vi "test Data Width 1 to 64.vi"(8 "error in (no error)":errorcluster, 11 "TestCase in":refnum<class "BCD.lvclass">) -> (0 "error out":errorcluster, 3 "TestCase out":refnum<class "BCD.lvclass">)   [LabVIEW 2027, in "BCD.lvclass"]
uses:
  BCD.lvclass
  080c8e86-f0ef-40bb-bb78-ec3bfa871640.vi
  0459340d-2ef3-43cd-ac4e-b003521538f2.vi
  Source/Get Bits Per Digit from Base.vi
  C:/Program Files/National Instruments/LabVIEW 2027/vi.lib/addons/_JKI Toolkits/VI Tester/TestCase.llb/TestCase.lvclass
  <vilib>/addons/_JKI Toolkits/VI Tester/TestCase.llb/TestCase.lvclass
panel:
  out "BCD encoded value":bool[](array[boolean])
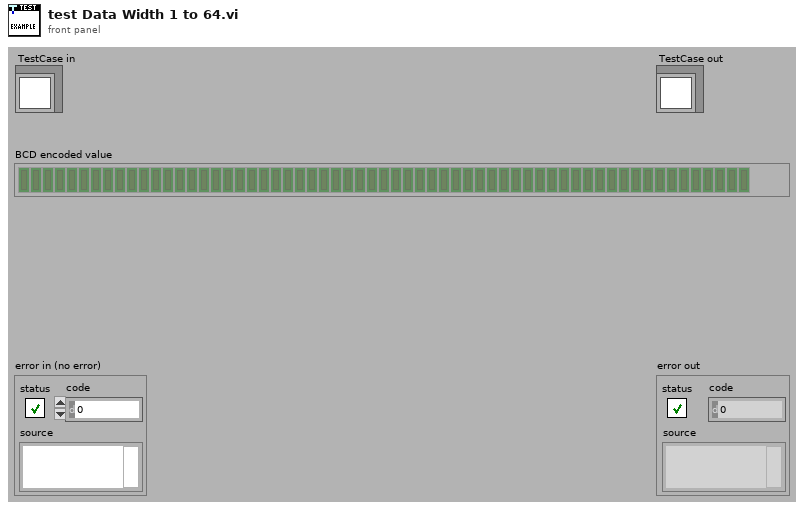
[diagram p1: front panel]
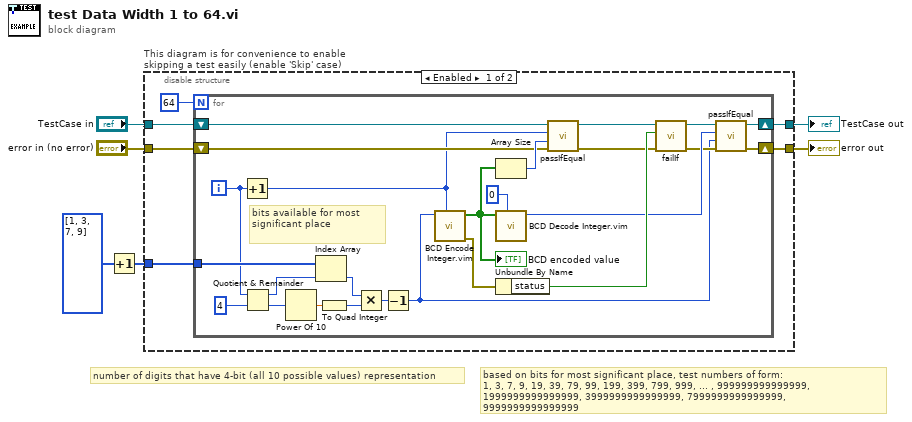
[diagram p0: block diagram]
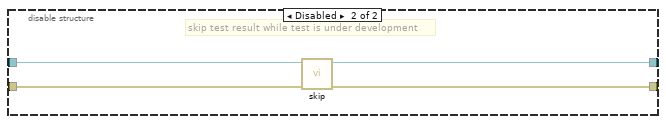
[diagram p2: hidden frame]
diagram:
  # "based on bits for most significant place, test numbers of form:\n1, 3, 7, 9, 19, 39, 79, 99, 199, 399, 799, 999, ... , 999999999999999, \n1999999999999999, 3999999999999999, 7999999999999999, 9999999999999999"
  # "number of digits that have 4-bit (all 10 possible values) representation"
  n1 = Increment(x=i64[] [1, 3, 7, 9]) -> (x+1=w1:i64[])
  n2 = disable-structure "This diagram is for convenience to enable skipping a test easily (enable 'Skip' case)" shown="Enabled" {
    disable-tunnel: "TestCase in" -> [w12 w41]
    disable-tunnel: [w10 w39] -> w3
    disable-tunnel: [w9 w40] -> w5
    disable-tunnel: "error in (no error)" -> [w11 w38]
    disable-tunnel: w1 -> [w7 _]
    frame Enabled {
      n3 = for {
        N: 64 -> [_]
        shift-right: [w25] -> w10
        shift-left: w12 -> [w32]
        shift-right: [w26] -> w9
        shift-left: w11 -> [w31]
        tunnel: w7 -> [w17]
        i -> [w16]
        # "bits available for most significant place"
        n4 = Increment(x=w16) -> (x+1=w15:i32)
        n5 = Quotient & Remainder(x=w16, y=4) -> (x-y*floor(x/y)=w19:i32, floor(x/y)=w22:i32)
        n6 = Power Of 10(x=w22) -> (10^x=w21:dbl)
        n7 = Index Array(array=w17, index=w19) -> (element=w20:i64)
        n8 = To Quad Integer(1:w21) -> (0:w23:i64)
        n9 = Multiply(x=w20, y=w23) -> (x*y=w24:i64)
        n10 = Decrement(x=w24) -> (x-1=w14:i64)
        n11 = call "BCD Encode Integer.vim"("data size (bits)"=w15, "integer"=w14) -> ("error out"=w36:errorcluster, "BCD encoded value"=w34:bool[])  [unwired: 8 in]
        "BCD encoded value" <- w34
        n12 = Array Size(array=w34) -> (size(s)=w35:i32)
        n13 = call "BCD Decode Integer.vim"("expected value and type"=i64 0, "BCD encoded value"=w34) -> ("integer"=w33:i64)  [unwired: 9 in]
        n14 = Unbundle By Name(w36) -> ("status"=w37:bool)
        n15 = call-dynamic "passIfEqual.vi"("error in (no error)"=w31, "y"=w35, "x"=w15, "TestCase in"=w32) -> ("error out"=w29:errorcluster, "TestCase out"=w30:refnum<class "BCD.lvclass">)  [unwired: 6 in]
        n16 = call-dynamic "failIf.vi"("error in (no error)"=w29, "fail"=w37, "TestCase in"=w30) -> ("error out"=w27:errorcluster, "TestCase out"=w28:refnum<class "BCD.lvclass">)  [unwired: 7 in]
        n17 = call-dynamic "passIfEqual.vi"("error in (no error)"=w27, "y"=w14, "x"=w33, "TestCase in"=w28) -> ("error out"=w26:errorcluster, "TestCase out"=w25:refnum<class "BCD.lvclass">)  [unwired: 6 in]
      }
    }
    frame Disabled {
      # "skip test result while test is under development"
      n18 = call <vilib>:"skip.vi"("error in (no error)"=w38, "TestCase in"=w41) -> ("error out"=w40:errorcluster, "TestCase out"=w39:refnum<class "BCD.lvclass">)  [unwired: 8 in]
    }
  }
  "error out" <- w5
  "TestCase out" <- w3
